vi "Clear Globals.vi"   [LabVIEW 2015]
uses:
  GlobalSender.vi
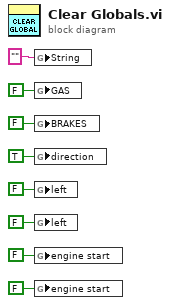
[diagram p0: block diagram]
diagram:
  n1 = global write "GlobalSender.vi" "String"("" ("String")) -> ()
  n2 = global write "GlobalSender.vi" "GAS"(FALSE ("GAS")) -> ()
  n3 = global write "GlobalSender.vi" "BRAKES"(FALSE ("BRAKES")) -> ()
  n4 = global write "GlobalSender.vi" "direction"(TRUE ("BRAKES")) -> ()
  n5 = global write "GlobalSender.vi" "left"(FALSE ("left")) -> ()
  n6 = global write "GlobalSender.vi" "left"(FALSE ("left")) -> ()
  n7 = global write "GlobalSender.vi" "engine start"(FALSE ("left")) -> ()
  n8 = global write "GlobalSender.vi" "engine start"(FALSE ("left")) -> ()
